vi "bus system link.vi"() -> ()   [LabVIEW 2019]
uses:
  Program Files (x86)/National Instruments/LabVIEW 2019/project/EN1Course-master (12)/EN1Course-master/_Subs/SystemLink/SL_Subs/SL_XControl.xctl
  Program Files (x86)/National Instruments/LabVIEW 2019/project/EN1Course-master (12)/EN1Course-master/_Subs/SystemLink/SL_Subs/SystemLink_Write_String.vi
  <vilib>/httpClient/LabVIEWHTTPClient.lvlib
panel:
  in  "SystemLink Tag":T1(xcontrol)={"Tag"="true96", "Type"="STRING", "Data"=""}
  in  "96":T1(xcontrol)={"Tag"="true94", "Type"="STRING", "Data"="03 minute(s), 44 second(s)"}
  in  "94":T1(xcontrol)={"Tag"="true94", "Type"="STRING", "Data"="03 minute(s), 44 second(s)"}
  out "94 bus":string="02 minute(s), 57 second(s)"
  in  "cat fact 2":T1(xcontrol)={"Tag"="cat", "Type"="STRING", "Data"=""}
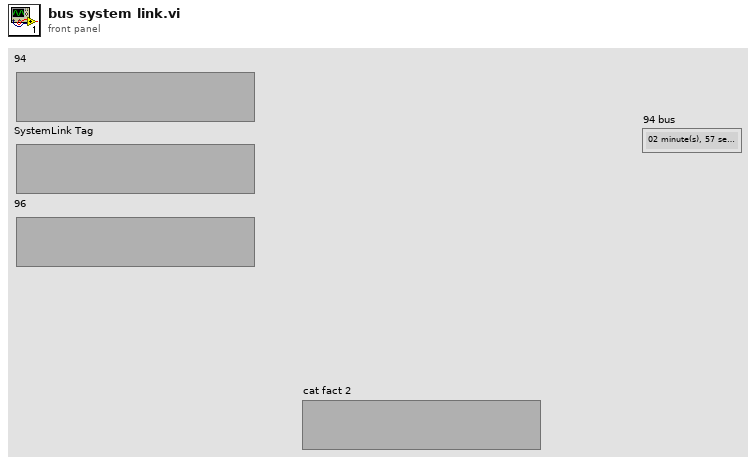
[diagram p1: front panel]
types:
  T1 = cluster{"Tag":string, "Type":string, "Data":string}
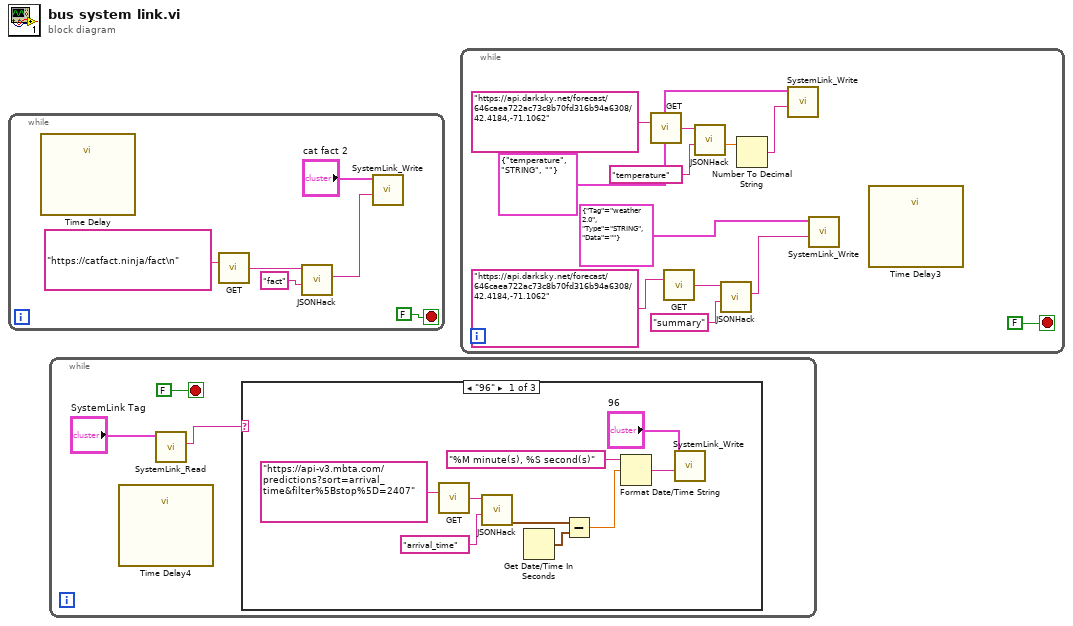
[diagram p0: block diagram]
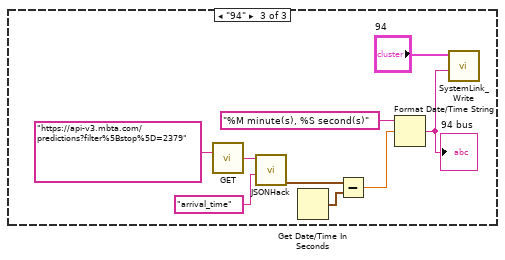
[diagram p3: hidden frame]
diagram:
  n1 = while {
    stop <- FALSE stop-if-true
    n2 = call "Time Delay"() -> ()  [unwired: 11 in, 1 out]
    n3 = call <vilib>:"GET.vi"("url"="https://catfact.ninja/fact\n") -> ("body"=w4:string)  [unwired: 11 in, 3 out]
    n4 = call "JSONHack.vi"("search name"="fact", "JSON in"=w4) -> ("Property (str)"=w2:string)  [unwired: 6 in, 3 out]
    n5 = call-poly "SystemLink_Write.vi"("String"=w2, "SL_XControl"="cat fact 2") -> ()  [unwired: 10 in]
  }
  n6 = while {
    stop <- FALSE stop-if-true
    n7 = call "Time Delay4"() -> ()  [unwired: 11 in, 1 out]
    n8 = call "SystemLink_Read.vi"("SystemLink Tag"="SystemLink Tag") -> ("value"=w9:string)  [unwired: 8 in, 2 out]
    n9 = case shown="\"96\"" w9 {
      frame "96" {
        n10 = call <vilib>:"GET.vi"("url"="https://api-v3.mbta.com/predictions?sort=arrival_time&filter%5Bstop%5D=2407") -> ("body"=w14:string)  [unwired: 11 in, 3 out]
        n11 = call "JSONHack.vi"("search name"="arrival_time", "JSON in"=w14) -> ("Property (time stamp)"=w12:timestamp)  [unwired: 6 in, 3 out]
        n12 = Get Date/Time In Seconds() -> (seconds since 1Jan1904=w17:timestamp)
        n13 = Subtract(x=w12, y=w17) -> (x-y=w18:dbl)
        n14 = Format Date/Time String(time format string (%c)="%M minute(s), %S second(s)", seconds (now)=w18) -> (date/time string=w11:string)  [unwired: 1 in]
        n15 = call-poly "SystemLink_Write.vi"("String"=w11, "SL_XControl"="96") -> ()  [unwired: 10 in]
      }
      frame Default {
      }
      frame "94" {
        n16 = call <vilib>:"GET.vi"("url"="https://api-v3.mbta.com/predictions?filter%5Bstop%5D=2379") -> ("body"=w23:string)  [unwired: 11 in, 3 out]
        n17 = call "JSONHack.vi"("search name"="arrival_time", "JSON in"=w23) -> ("Property (time stamp)"=w21:timestamp)  [unwired: 6 in, 3 out]
        n18 = Get Date/Time In Seconds() -> (seconds since 1Jan1904=w26:timestamp)
        n19 = Subtract(x=w21, y=w26) -> (x-y=w27:dbl)
        n20 = Format Date/Time String(time format string (%c)="%M minute(s), %S second(s)", seconds (now)=w27) -> (date/time string=w20:string)  [unwired: 1 in]
        "94 bus" <- w20
        n21 = call-poly "SystemLink_Write.vi"("String"=w20, "SL_XControl"="94") -> ()  [unwired: 10 in]
      }
    }
  }
  n22 = while {
    stop <- FALSE stop-if-true
    n23 = call <vilib>:"GET.vi"("url"="https://api.darksky.net/forecast/646caea722ac73c8b70fd316b94a6308/42.4184,-71.1062") -> ("body"=w32:string)  [unwired: 11 in, 3 out]
    n24 = call <vilib>:"GET.vi"("url"="https://api.darksky.net/forecast/646caea722ac73c8b70fd316b94a6308/42.4184,-71.1062") -> ("body"=w37:string)  [unwired: 11 in, 3 out]
    n25 = call "JSONHack.vi"("search name"="temperature", "JSON in"=w32) -> ("Property (num)"=w30:dbl)  [unwired: 6 in, 3 out]
    n26 = call "JSONHack.vi"("search name"="summary", "JSON in"=w37) -> ("Property (str)"=w35:string)  [unwired: 6 in, 3 out]
    n27 = Number To Decimal String(number=w30) -> (decimal integer string=w29:string)  [unwired: 1 in]
    n28 = call-poly "SystemLink_Write.vi"("String"=w29, "SL_XControl"=T1 {"Tag"="temperature", "Type"="STRING", "Data"=""} ("temperature")) -> ()  [unwired: 10 in]
    n29 = call-poly "SystemLink_Write.vi"("String"=w35, "SL_XControl"=T1 {"Tag"="weather 2.0", "Type"="STRING", "Data"=""} ("weather summary")) -> ()  [unwired: 10 in]
    n30 = call "Time Delay3"() -> ()  [unwired: 11 in, 1 out]
  }
